vi "ElevatorPositionConfigUI .vi"() -> (1 "Confirmed?":bool, 3 "ElevatorPositionConfiguration":T1)   [LabVIEW 2021]
uses:
  TypeDefs/ElevatorPositionConfiguration.ctl
panel:
  in  "Cancel":bool
  in  "Confirm button":bool
  in  "ServomotorRotates":bool caption="Do you wish servomotor rotates along the elevator movement?"
  in  "Start Position":dbl
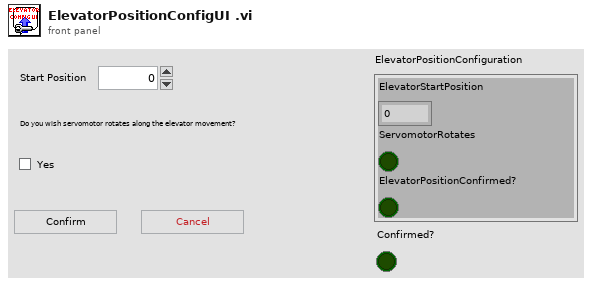
[diagram p1: front panel]
types:
  T1 = typedef "ElevatorPositionConfiguration.ctl" = cluster{"ElevatorStartPosition":dbl, "ServomotorRotates":bool, "ElevatorPositionConfirmed?":bool}
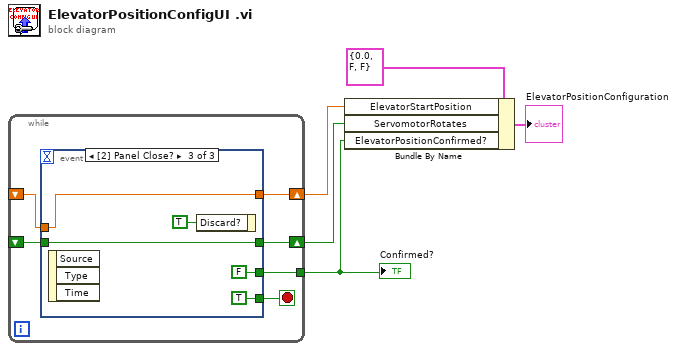
[diagram p0: block diagram]
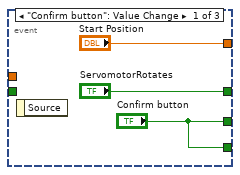
[diagram p2: hidden frame]
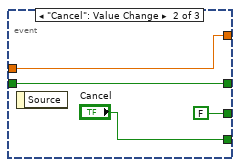
[diagram p3: hidden frame]
diagram:
  n1 = while {
    shift-right: [w11] -> w5
    shift-left: _ -> [w9]
    shift-right: [w10] -> w4
    shift-left: _ -> [w8]
    tunnel: [w7] -> w1
    stop <- w6 stop-if-true
    n2 = event shown="[2] Panel Close?" {
      selector: _ -> [_ _ _]
      dyn-events: _ -> [_ _ _]
      timeout: _ -> [_ _ _]
      tunnel: ["Start Position" w18 w20] -> w11
      tunnel: ["ServomotorRotates" w16 w19] -> w10
      tunnel: w9 -> [_ w18 w20]
      tunnel: w8 -> [_ w16 w19]
      tunnel: ["Confirm button" FALSE ("Confirm button") FALSE ("Confirm button")] -> w7
      tunnel: ["Confirm button" "Cancel" TRUE ("Cancel")] -> w6
      event "Confirm button": Value Change {
        n3 = event-data() -> ()  [unwired: 1 in, 1 out]
      }
      event "Cancel": Value Change {
        n4 = event-data() -> ()  [unwired: 1 in, 1 out]
      }
      event Panel Close? {
        n5 = event-data() -> ()  [unwired: 1 in, 3 out]
        n6 = event-data("Discard?"=TRUE) -> ()  [unwired: 1 in, 1 out]
      }
    }
  }
  "Confirmed?" <- w1
  n7 = Bundle By Name(cluster=T1 {"ElevatorStartPosition"=0.0, "ServomotorRotates"=FALSE, "ElevatorPositionConfirmed?"=FALSE} ("ElevatorPositionConfiguration"), "ElevatorStartPosition"=w5, "ServomotorRotates"=w4, "ElevatorPositionConfirmed?"=w1) -> (→"ElevatorPositionConfiguration":T1)
